vi "MODBUS_SALICRU.vi"() -> ()   [LabVIEW 2024]
uses:
  <vilib>/Modbus/master/Create Master Instance (TCP).vi
  <vilib>/Modbus/master/Modbus Master.lvclass
  SALICRU_MODBUS.lvlib
panel:
  out "x/y":dbl
  in  "stop":bool
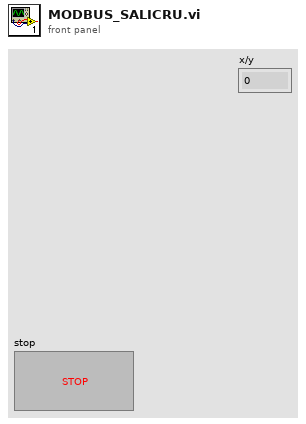
[diagram p1: front panel]
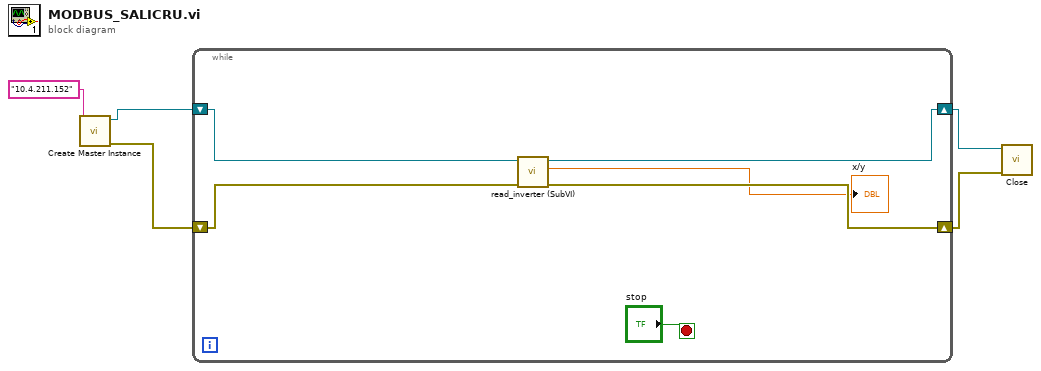
[diagram p0: block diagram]
diagram:
  n1 = call-poly <vilib>:"Create Master Instance.vi"("address"="10.4.211.152") -> ("error out"=w4:errorcluster, "TCP master instance"=w5:refnum<class "Modbus Master.lvclass">)  [unwired: 9 in]
  n2 = while {
    shift-right: [w8] -> w3
    shift-left: w5 -> [w11]
    shift-right: [w9] -> w2
    shift-left: w4 -> [w10]
    stop <- "stop" stop-if-true
    n3 = call "read_inverter (SubVI).vi"("error in (no error)"=w10, "Modbus Master in"=w11) -> ("error out"=w9:errorcluster, "x/y"=→"x/y":dbl, "Modbus Master out"=w8:refnum<class "Modbus Master.lvclass">)  [unwired: 7 in]
  }
  n4 = call-dynamic "Close.vi"("error in (no error)"=w2, "Modbus master in"=w3) -> ()  [unwired: 9 in, 1 out]
